vi "IviAcquisitionToProperty.vi"(8 "error in (no error)":errorcluster, 11 "IVI_Class.lvclass":refnum<class "IVI_Class.lvclass">) -> (0 "error out":errorcluster, 3 "IVI_Class.lvclass":refnum<class "IVI_Class.lvclass">)   [LabVIEW 2018, in "ScopePlugins.lvlib" / "IVI_Class.lvclass"]
doc: "Reads IVI Scope Acquisition properties and writes them into the Scope class Acquisition Properties"
uses:
  IVI_Class.lvclass
  F:/Projects/ICDAS/NistPluggableModules/Scope/ScopePlugins/ScopePluginBaseClass/ScopePluginsBase.lvclass
  ScopePluginBaseClass/ScopePluginsBase.lvclass/ScopePluginsBase.ctl
  ScopePluginBaseClass/Typedefs/HorizontalSettings.ctl
  ScopePluginBaseClass/Accessors/Read Channels.vi
  ScopePluginBaseClass/ScopePluginsBase.lvclass
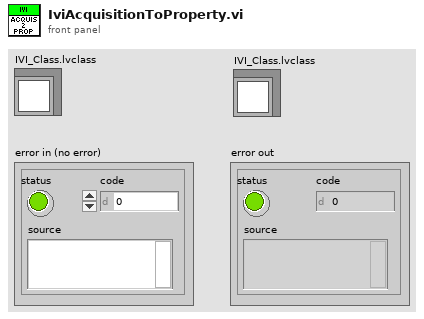
[diagram p1: front panel]
types:
  T1 = typedef "ScopePlugins.lvlib/ScopePluginsBase.lvclass/HorizontalSettings.ctl" = cluster{"Continuous":bool, "EnableAveraging":bool, "Number Averages":i32, "Measurement Timeout":dbl, "Min Record Length":i32, "Min Sample Rate":dbl, "Enforce Realtime":bool, "Sampling Mode ":enum16{"Real Time", "Equivalent Time", "Segment", "Real Time Peak Detect", "Real Time High Resolution", "Peak Detect Segment", "High Resolution Segment"}, "Interpolation":enum16{"No Interpolation", "sin(x)/x", "linear", "1 Point sin(x)/x", "2 Point sin(x)/x", "4 Point sin(x)/x", "8 Point sin(x)/x", "16 Point sin(x)/x"}, "Type":enum16{"Normal", "PeakDetect", "HighRes", "Envelope", "Average"}, "StartTime":dbl, "Time Per Record":dbl, "Number of Points Minimum":i32, "Measurement Name":string, "Measurement RefreshTime (ms)":u32}
  T2 = typedef "ScopePlugins.lvlib/ScopePluginsBase.lvclass/ChannelSetting(s).ctl" = cluster{"Number of Channels":i32, "Channel(s)":cluster{"Enabled":bool, "Instrument Handle":string, "Channel Name":string, "Maximum Input Frequency":dbl, "Verticle Settings":cluster{"Vertical Range":dbl, "Vertical Offset":dbl, "Probe Attenuation":dbl, "Vertical Coupling":i32}, "Connected":bool, "Input Impedance":dbl, "IO Type Instrument Handle":refnum<k15>}[]}
  T3 = cluster{"Enabled":bool, "Instrument Handle":string, "Channel Name":string, "Maximum Input Frequency":dbl, "Verticle Settings":cluster{"Vertical Range":dbl, "Vertical Offset":dbl, "Probe Attenuation":dbl, "Vertical Coupling":i32}, "Connected":bool, "Input Impedance":dbl, "IO Type Instrument Handle":refnum<k15>}[]
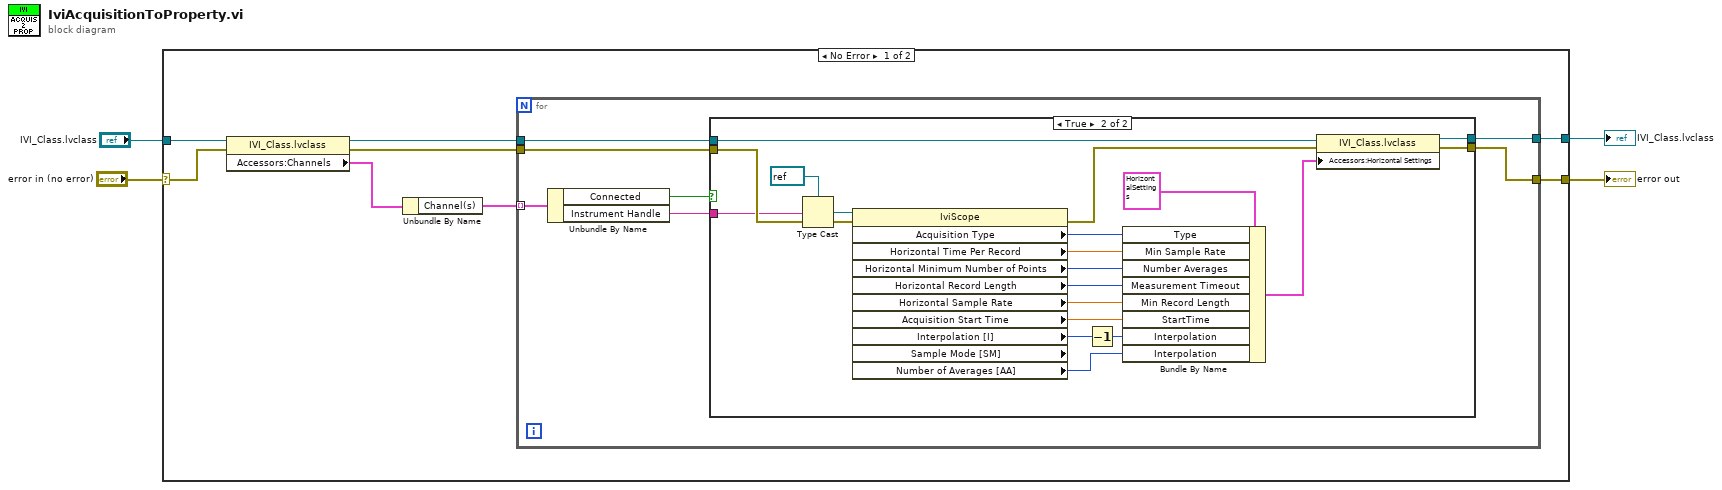
[diagram p0: block diagram]
diagram:
  n1 = case shown="No Error" "error in (no error)" {
    selector: "error in (no error)" -> [w9 w41]
    tunnel: "IVI_Class.lvclass" -> [w12 w42]
    tunnel: [w10 w42] -> w3
    tunnel: [w7 w41] -> w1
    frame No Error {
      n2 = property class="IVI_Class.lvclass"(reference=w12, error in=w9) -> (reference out=w11:refnum<class "IVI_Class.lvclass">, error out=w8:errorcluster, "Accessors:Channels"=w6:T2)
      n3 = Unbundle By Name(w6) -> ("Channel(s)"=w5:T3)
      n4 = for {
        tunnel: w11 -> [w19]
        tunnel: [w18] -> w10
        tunnel: w5 -> [w15] mode=indexing
        tunnel: w8 -> [w17]
        tunnel: [w16] -> w7
        n5 = Unbundle By Name(w15) -> ("Connected"=w14:bool, "Instrument Handle"=w13:string)
        n6 = case shown="True" w14 {
          tunnel: w19 -> [w21 w38]
          tunnel: [w21 w35] -> w18
          tunnel: w17 -> [w20 w34]
          tunnel: [w20 w32] -> w16
          tunnel: w13 -> [_ w22]
          frame False {
          }
          frame True {
            n7 = Type Cast(type=refnum<k15> refnum ("reference out"), x=w22) -> (*(type *) &x=w39:refnum<k15>)
            n8 = property class="IviScope" props=["Acquisition Type", "Horizontal Time Per Record", "Horizontal Minimum Number of Points", "Horizontal Record Length", "Horizontal Sample Rate", "Acquisition Start Time", "Interpolation [I]", "Sample Mode [SM]", "Number of Averages [AA]"](reference=w39, error in=w34) -> (error out=w33:errorcluster, "Acquisition Type"=w37:i32, "Horizontal Time Per Record"=w31:dbl, "Horizontal Minimum Number of Points"=w30:i32, "Horizontal Record Length"=w29:i32, "Horizontal Sample Rate"=w28:dbl, "Acquisition Start Time"=w27:dbl, "Interpolation [I]"=w26:i32, "Number of Averages [AA]"=w25:i32)  [unwired: 2 out]
            n9 = Decrement(x=w26) -> (x-1=w24:i32)
            n10 = Bundle By Name(cluster=T1 {"Continuous"=FALSE, "EnableAveraging"=FALSE, "Number Averages"=0, "Measurement Timeout"=0.0, "Min Record Length"=1000, "Min Sample Rate"=10000000.0, "Enforce Realtime"=TRUE, "Sampling Mode "=enum."Real Time", "Interpolation"=enum."No Interpolation", "Type"=enum."Normal", "StartTime"=0.0, "Time Per Record"=0.0, "Number of Points Minimum"=0, "Measurement Name"="Sensor.RoomAlert0", "Measurement RefreshTime (ms)"=1000} ("Horizontal Settings"), "Type"=w37, "Min Sample Rate"=w31, "Number Averages"=w30, "Measurement Timeout"=w29, "Min Record Length"=w28, "StartTime"=w27, "Interpolation"=w24, "Interpolation"=w25) -> (w36:T1)
            n11 = property class="IVI_Class.lvclass"(reference=w38, error in=w33, "Accessors:Horizontal Settings"=w36) -> (reference out=w35:refnum<class "IVI_Class.lvclass">, error out=w32:errorcluster)
          }
        }
      }
    }
    frame Error {
    }
  }
  "IVI_Class.lvclass" <- w3
  "error out" <- w1
